vi "Search.vi"(6 "Index in":i32=-1, 7 "Composite Object":refnum<class "CConfig Object.lvclass">, 8 "error in (no error)":errorcluster, 11 "Find Query in":refnum<class "Match Query.lvclass">) -> (0 "error out":errorcluster, 2 "empty?":bool, 3 "Find Query out":refnum<class "Match Query.lvclass">, 5 "Composite Object":refnum<class "CConfig Object.lvclass">)   [LabVIEW 2013, in "Match Query.lvclass"]
doc: "Copyright 2018, Carya Automatisering, Wiebe Walstra."
uses:
  Match Query.lvclass
  CConfig Object.lvclass
  Match Query.lvclass/Match Query.ctl
  Data.ctl
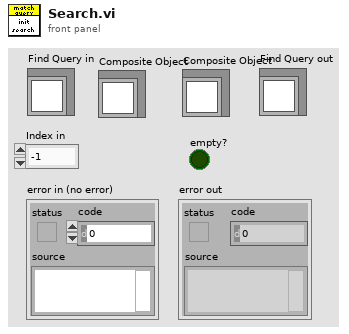
[diagram p1: front panel]
types:
  T1 = typedef "CConfig Object.lvclass/Data.ctl" = enum16{"pre", "name", "middle", "value", "post", "newline", "persistant", "tagged", "type"}
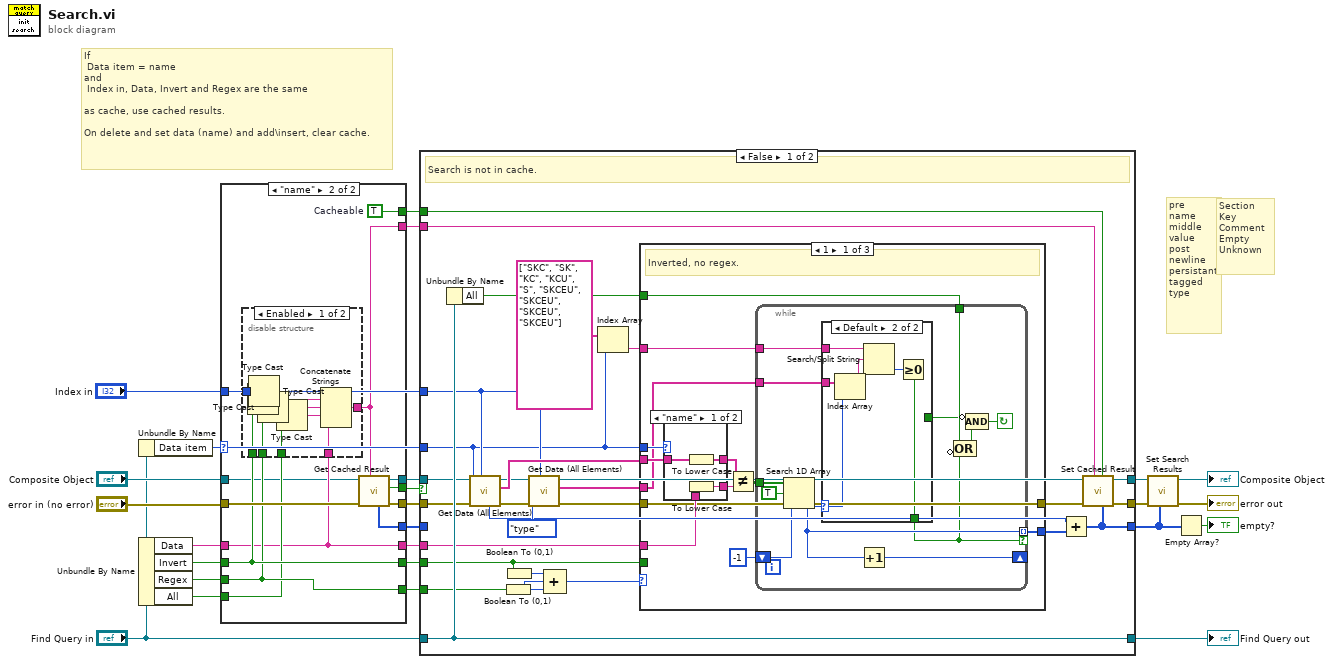
[diagram p0: block diagram]
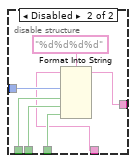
[diagram p3: hidden frame]
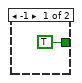
[diagram p5: hidden frame]
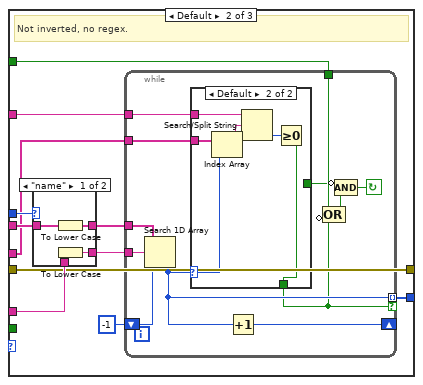
[diagram p6: hidden frame]
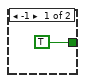
[diagram p8: hidden frame]
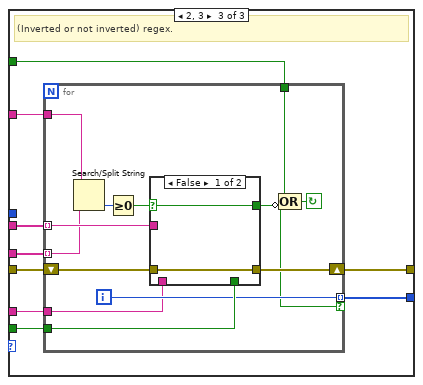
[diagram p9: hidden frame]
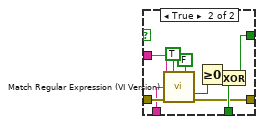
[diagram p10: hidden frame]
diagram:
  # "pre\nname\nmiddle\nvalue\npost \nnewline\npersistant\ntagged\ntype"
  # "Section\nKey\nComment\nEmpty\nUnknown"
  # "If \n Data item = name\nand\n Index in, Data, Invert and Regex are the same\n\nas cache, use cached results.\n\nOn delete and set data (name) and add\\insert, clear cache."
  n1 = Unbundle By Name("Find Query in") -> ("Data item"=w9:T1)
  n2 = Unbundle By Name("Find Query in") -> ("Data"=w7:string, "Invert"=w5:bool, "Regex"=w3:bool, "All"=w2:bool)
  n3 = case shown="\"name\"" w9 {
    tunnel: "error in (no error)" -> [w29 w43]
    tunnel: "Index in" -> [_ w39]
    tunnel: [w29 w42] -> w18
    tunnel: "Composite Object" -> [w30 w33]
    tunnel: [w30 w32] -> w16
    tunnel: [_ w31] -> w15
    tunnel: [_ w41] -> w12
    tunnel: [_ w40] -> w11
    tunnel: [_ w34] -> w10
    tunnel: [w28 w35] -> w8
    tunnel: w7 -> [w28 w35]
    tunnel: [w27 w38] -> w6
    tunnel: w5 -> [w27 w38]
    tunnel: [w26 w37] -> w4
    tunnel: w3 -> [w26 w37]
    tunnel: w2 -> [_ w36]
    frame Default {
    }
    frame "name" {
      w40 = TRUE  # Cacheable
      n4 = disable-structure shown="Enabled" {
        disable-tunnel: w39 -> [w53 w60]
        disable-tunnel: w38 -> [w52 w59]
        disable-tunnel: w37 -> [w51 w58]
        disable-tunnel: w36 -> [w50 w57]
        disable-tunnel: w35 -> [w45 w56]
        disable-tunnel: [w44 w54] -> w34
        frame Enabled {
          n5 = Type Cast(x=w52) -> (*(type *) &x=w48:string)  [unwired: 1 in]
          n6 = Type Cast(x=w53) -> (*(type *) &x=w49:string)  [unwired: 1 in]
          n7 = Type Cast(x=w51) -> (*(type *) &x=w47:string)  [unwired: 1 in]
          n8 = Type Cast(x=w50) -> (*(type *) &x=w46:string)  [unwired: 1 in]
          n9 = Concatenate Strings(w49, w48, w47, w46, w45) -> (w44:string)
        }
        frame Disabled {
          n10 = Format Into String(format string="%d%d%d%d", initial string=w56, w60, w59, w58, w57) -> (resulting string=w54:string)  [unwired: 1 in, 1 out]
        }
      }
      n11 = call-dynamic "Get Cached Result.vi"("Cache string"=w34, "error in (no error)"=w43, "Composite Object in"=w33) -> ("error out"=w42:errorcluster, "Cached?"=w31:bool, "Composite Object out"=w32:refnum<class "CConfig Object.lvclass">, "Cached results"=w41:i32[])  [unwired: 5 in]
    }
  }
  n12 = case shown="False" w15 {
    tunnel: [w83 w199] -> w24
    tunnel: [w61 w200] -> w22
    tunnel: [w80 w198] -> w14
    tunnel: "Index in" -> [w66 _]
    tunnel: "Find Query in" -> [w84 w197]
    tunnel: w18 -> [w78 w199]
    tunnel: w16 -> [w79 w200]
    tunnel: w12 -> [_ w198]
    tunnel: [w84 w197] -> w13
    tunnel: w11 -> [w81 _]
    tunnel: w10 -> [w82 _]
    tunnel: w9 -> [w64 _]
    tunnel: w8 -> [w76 _]
    tunnel: w6 -> [w75 _]
    tunnel: w4 -> [w74 _]
    frame False {
      # "Search is not in cache."
      n13 = Unbundle By Name(w84) -> ("All"=w85:bool)
      n14 = call "Get Data (All Elements).vi"("Start index [0]"=w66, "error in (no error)"=w78, "Data [name]"=w64, "Composite Object in"=w79) -> ("error out"=w73:errorcluster, "Data"=w77:string[], "Composite Object out"=w71:refnum<class "CConfig Object.lvclass">, "First part"=w63:i32)  [unwired: 4 in]
      n15 = Boolean To (0,1)(Boolean=w74) -> (0, 1=w88:i16)
      n16 = Boolean To (0,1)(Boolean=w75) -> (0, 1=w87:i16)
      n17 = call "Get Data (All Elements).vi"("Start index [0]"=w66, "error in (no error)"=w73, "Data [name]"=Data."type", "Composite Object in"=w71) -> ("error out"=w72:errorcluster, "Data"=w69:string[], "Composite Object out"=w62:refnum<class "CConfig Object.lvclass">)  [unwired: 4 in, 1 out]
      n18 = Compound Arithmetic op=ADD(w87, w88, w88) -> (w89:i16)
      n19 = Index Array(array=string[] ["SKC", "SK", "KC", "KCU", "S", "SKCEU", "SKCEU", "SKCEU", "SKCEU"], index=w64) -> (element=w65:string)
      n20 = case shown="1" w89 {
        tunnel: w64 -> [w92 w135 _]
        tunnel: w77 -> [w101 w137 w167]
        tunnel: w76 -> [w100 w136 w171]
        tunnel: w72 -> [w96 w134 w170]
        tunnel: [w96 w134 w169] -> w68
        tunnel: w75 -> [_ _ w168]
        tunnel: [w94 w132 w166] -> w86
        tunnel: w85 -> [w93 w131 w165]
        tunnel: w69 -> [w91 w128 w164]
        tunnel: w65 -> [w90 w127 w163]
        frame 1 {
          # "Inverted, no regex."
          n21 = case shown="\"name\"" w92 {
            tunnel: w101 -> [w105 w107]
            tunnel: [w102 w107] -> w99
            tunnel: w100 -> [w104 w106]
            tunnel: [w103 w106] -> w98
            frame "name" {
              n22 = To Lower Case(string=w105) -> (all lower case string=w102:string[])
              n23 = To Lower Case(string=w104) -> (all lower case string=w103:string)
            }
            frame Default {
            }
          }
          n24 = Not Equal?(x=w99, y=w98) -> (x != y?=w97:bool[])
          n25 = while {
            tunnel: w97 -> [w118]
            shift-right: [w116] -> _
            shift-left: -1 ("index of element") -> [w119]
            tunnel: [w115] -> w94 mode=indexing if=w110
            tunnel: w93 -> [w114]
            tunnel: w91 -> [w109]
            tunnel: w90 -> [w108]
            stop <- w111 continue-if-true
            n26 = Search 1D Array(1D array=w118, element=TRUE, start index (0)=w119) -> (index of element=w115:i32)
            n27 = case shown="Default" w115 {
              selector: w115 -> [_ w125]
              tunnel: [_ w121] -> w110
              tunnel: [TRUE _] -> w113
              tunnel: w109 -> [_ w126]
              tunnel: w108 -> [_ w123]
              frame -1 {
              }
              frame Default {
                n28 = Index Array(array=w126, index=w125) -> (element=w122:string)
                n29 = Search/Split String(string=w123, search string/char (-)=w122) -> (offset of match=w124:i32)  [unwired: 1 in, 2 out]
                n30 = Greater Or Equal To 0?(x=w124) -> (x >= 0?=w121:bool)
              }
            }
            n31 = Increment(x=w115) -> (x+1=w116:i32)
            n32 = Compound Arithmetic op=OR(w114, invert w110) -> (w112:bool)
            n33 = Compound Arithmetic op=AND(invert w113, w112) -> (w111:bool)
          }
        }
        frame Default {
          # "Not inverted, no regex."
          n34 = case shown="\"name\"" w135 {
            tunnel: w137 -> [w141 w143]
            tunnel: [w138 w143] -> w130
            tunnel: w136 -> [w140 w142]
            tunnel: [w139 w142] -> w129
            frame "name" {
              n35 = To Lower Case(string=w141) -> (all lower case string=w138:string[])
              n36 = To Lower Case(string=w140) -> (all lower case string=w139:string)
            }
            frame Default {
            }
          }
          n37 = while {
            tunnel: w130 -> [w154]
            shift-right: [w153] -> _
            shift-left: -1 ("index of element") -> [w155]
            tunnel: [w152] -> w132 mode=indexing if=w147
            tunnel: w131 -> [w151]
            tunnel: w129 -> [w146]
            tunnel: w128 -> [w145]
            tunnel: w127 -> [w144]
            stop <- w148 continue-if-true
            n38 = Search 1D Array(1D array=w154, element=w146, start index (0)=w155) -> (index of element=w152:i32)
            n39 = case shown="Default" w152 {
              selector: w152 -> [_ w161]
              tunnel: [_ w157] -> w147
              tunnel: [TRUE _] -> w150
              tunnel: w145 -> [_ w162]
              tunnel: w144 -> [_ w159]
              frame -1 {
              }
              frame Default {
                n40 = Index Array(array=w162, index=w161) -> (element=w158:string)
                n41 = Search/Split String(string=w159, search string/char (-)=w158) -> (offset of match=w160:i32)  [unwired: 1 in, 2 out]
                n42 = Greater Or Equal To 0?(x=w160) -> (x >= 0?=w157:bool)
              }
            }
            n43 = Increment(x=w152) -> (x+1=w153:i32)
            n44 = Compound Arithmetic op=OR(w151, invert w147) -> (w149:bool)
            n45 = Compound Arithmetic op=AND(invert w150, w149) -> (w148:bool)
          }
        }
        frame 2, 3 {
          # "(Inverted or not inverted) regex."
          n46 = for {
            tunnel: w167 -> [w180] mode=indexing
            tunnel: w171 -> [w179]
            shift-right: [w177] -> w169
            shift-left: w170 -> [w178]
            tunnel: w168 -> [w184]
            tunnel: [w183] -> w166 mode=indexing if=w176
            tunnel: w165 -> [w181]
            tunnel: w164 -> [w173] mode=indexing
            tunnel: w163 -> [w174]
            i -> [w183]
            stop <- w182 continue-if-true
            n47 = Search/Split String(string=w174, search string/char (-)=w173) -> (offset of match=w175:i32)  [unwired: 1 in, 2 out]
            n48 = Greater Or Equal To 0?(x=w175) -> (x >= 0?=w172:bool)
            n49 = case shown="False" w172 {
              selector: w172 -> [w185 _]
              tunnel: w184 -> [_ w195]
              tunnel: w178 -> [w186 w194]
              tunnel: [w186 w193] -> w177
              tunnel: w180 -> [_ w190]
              tunnel: w179 -> [_ w189]
              tunnel: [w185 w187] -> w176
              frame False {
              }
              frame True {
                n50 = call "Match Regular Expression (VI Version).vi"("ignore case? (F)"=TRUE, "return results? (T)"=FALSE, "input string"=w190, "regular expression"=w189, "error in"=w194) -> ("offset past match"=w192:i32, "error out"=w193:errorcluster)  [unwired: 4 in, 5 out]
                n51 = Greater Or Equal To 0?(x=w192) -> (x >= 0?=w196:bool)
                n52 = Exclusive Or(1:w195, 2:w196) -> (0:w187:bool)
              }
            }
            n53 = Compound Arithmetic op=OR(w181, invert w176) -> (w182:bool)
          }
        }
      }
      n54 = Add(x=w63, y=w86) -> (x+y=w80:i32[])
      n55 = call-dynamic "Set Cached Result.vi"("Cached results"=w80, "Cacheable?"=w81, "Cache string"=w82, "error in (no error)"=w68, "Composite Object in"=w62) -> ("error out"=w83:errorcluster, "Composite Object out"=w61:refnum<class "CConfig Object.lvclass">)  [unwired: 5 in]
    }
    frame True {
      # "Search is cached."
    }
  }
  "Find Query out" <- w13
  n56 = call-dynamic "Set Search Results.vi"("Search results"=w14, "error in (no error)"=w24, "Composite Object in"=w22) -> ("error out"=→"error out":errorcluster, "Composite Object out"=→"Composite Object":refnum<class "CConfig Object.lvclass">)  [unwired: 7 in]
  n57 = Empty Array?(array=w14) -> (empty?=→"empty?":bool)
